vi "Get Database Information.vi"() -> ()   [LabVIEW 2013]
doc: "This example returns information contained in a database named LabVIEW.mdb located in the LabVIEW examples>>database directory. The information consists of the table names, column names, data types, and data sizes."
uses:
  Connection.llb/DB Tools Open Connec (Path).vi
  NI_Database_API_64.lvlib
panel:
  out "Database Information":string[][](table)
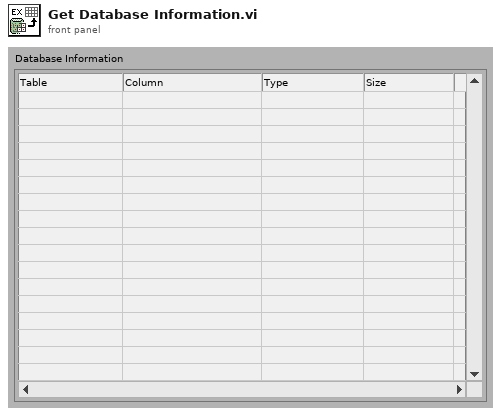
[diagram p1: front panel]
types:
  T1 = typedef "NI_Database_API_64.lvlib/Conn ObjectReference.ctl" = refnum<k1>
  T2 = typedef "NI_Database_API_64.lvlib/DB Tools DataTypes.ctl" = enum16{"String", "Long (I32)", "Single (SGL)", "Double (DBL)", "Date/Time", "Binary"}
  T3 = cluster{"name":string, "database data type":T2, "defined size":i32}[]
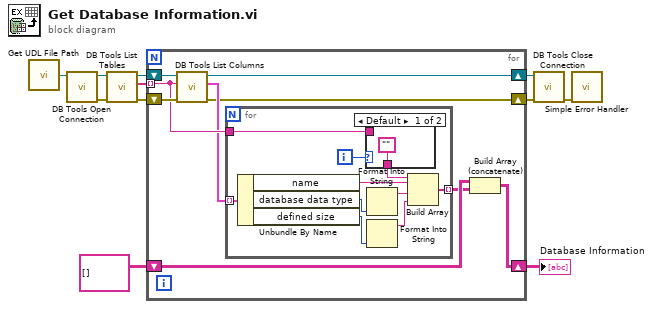
[diagram p0: block diagram]
diagram:
  n1 = call "Get UDL File Path.vi"() -> ("UDL file path"=w1:path)  [unwired: 1 in]
  n2 = call-poly "DB Tools Open Connection.vi"("connection information"=w1) -> ("error out"=w11:errorcluster, "connection reference"=w10:T1)  [unwired: 7 in]
  n3 = call "DB Tools List Tables.vi"("error in (no error)"=w11, "connection reference"=w10) -> ("error out"=w8:errorcluster, "tables"=w7:string[], "connection reference out"=w9:T1)  [unwired: 3 in]
  n4 = for {
    shift-right: [w16] -> w4
    shift-left: w8 -> [w20]
    tunnel: w7 -> [w18] mode=indexing
    shift-right: [w15] -> w6
    shift-left: string[][] [] -> [w14]
    shift-right: [w12] -> w3
    shift-left: w9 -> [w19]
    n5 = call "DB Tools List Columns.vi"("error in (no error)"=w20, "table"=w18, "connection reference"=w19) -> ("error out"=w16:errorcluster, "column information"=w17:T3, "connection reference out"=w12:T1)  [unwired: 1 in, 1 out]
    n6 = for {
      tunnel: w18 -> [w29]
      tunnel: w17 -> [w26] mode=indexing
      tunnel: [w28] -> w13 mode=indexing
      i -> [w30]
      n7 = Unbundle By Name(w26) -> ("name"=w25:string, "database data type"=w24:T2, "defined size"=w22:i32)
      n8 = case shown="Default" w30 {
        tunnel: w29 -> [_ w32]
        tunnel: ["" w32] -> w27
        frame Default {
        }
        frame 0 {
        }
      }
      n9 = Format Into String(w24) -> (resulting string=w23:string)  [unwired: 3 in, 1 out]
      n10 = Format Into String(w22) -> (resulting string=w21:string)  [unwired: 3 in, 1 out]
      n11 = Build Array(w27, w25, w23, w21) -> (w28:string[])
    }
    n12 = Build Array (concatenate)(w14, w13) -> (w15:string[][])
  }
  "Database Information" <- w6
  n13 = call "DB Tools Close Connection.vi"("error in (no error)"=w4, "connection reference"=w3) -> ("error out"=w2:errorcluster)  [unwired: 5 in]
  n14 = call <vilib>:"Simple Error Handler.vi"("error in (no error)"=w2) -> ()  [unwired: 4 in, 5 out]
